vi "Get 8-Byte Integer.vi"(11 "Bytes in":u8[](array[numeric])) -> (1 "8-Byte Integer":u64, 3 "Bytes out":u8[](array[numeric]))   [LabVIEW 2014, in "hse-db.lvlib" / "MySQL (TCP).lvlib"]
uses:
  MySQL (TCP).lvlib
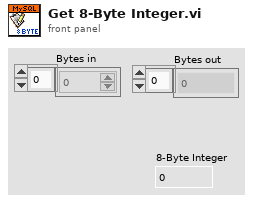
[diagram p1: front panel]
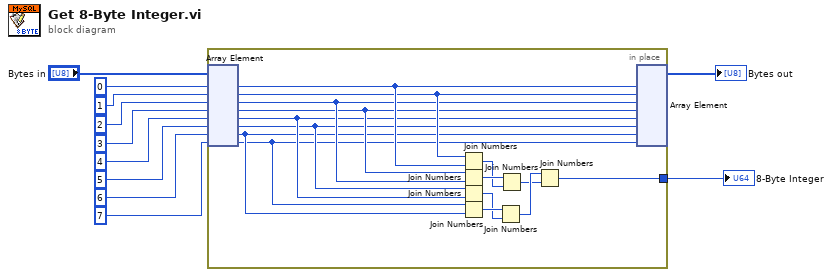
[diagram p0: block diagram]
diagram:
  n1 = in-place {
    in-place-border: [w26] -> w11
    n2 = in-place-array #1("Bytes in", 0, 1, 2, 3, 4, 5, 6, 7) -> (w19:u8, w18:u8, w17:u8, w16:u8, w15:u8, w14:u8, w13:u8, w12:u8)
    n3 = Join Numbers(hi=w18, lo=w19) -> ((hi.lo)=w20:u16)
    n4 = Join Numbers(hi=w16, lo=w17) -> ((hi.lo)=w21:u16)
    n5 = Join Numbers(hi=w14, lo=w15) -> ((hi.lo)=w22:u16)
    n6 = Join Numbers(hi=w12, lo=w13) -> ((hi.lo)=w23:u16)
    n7 = Join Numbers(hi=w23, lo=w22) -> ((hi.lo)=w25:u32)
    n8 = Join Numbers(hi=w21, lo=w20) -> ((hi.lo)=w24:u32)
    n9 = Join Numbers(hi=w25, lo=w24) -> ((hi.lo)=w26:u64)
    n10 = in-place-array #1(w19, w18, w17, w16, w15, w14, w13, w12) -> (→"Bytes out":u8[])  [unwired: 8 out]
  }
  "8-Byte Integer" <- w11
